vi "Default controls - load control values.vi"(8 "error in (no error)":errorcluster, 11 "path":path) -> (0 "error out":errorcluster, 3 "path to ini":path)   [LabVIEW 2020]
uses:
  Save-Load-Defaults.lvlib/Save-Load-Defaults.lvlib
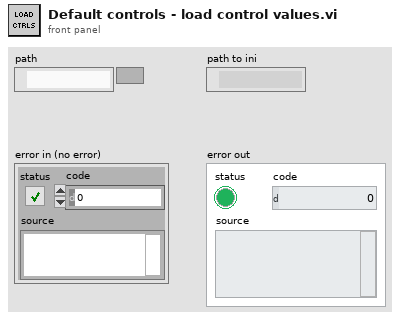
[diagram p1: front panel]
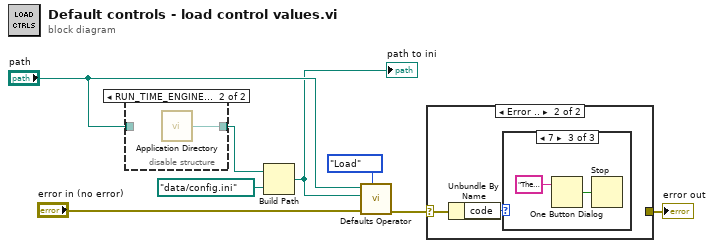
[diagram p0: block diagram]
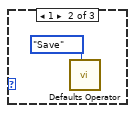
[diagram p4: hidden frame]
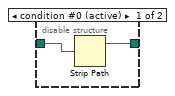
[diagram p5: hidden frame]
diagram:
  n1 = disable-structure shown="RUN_TIME_ENGINE==True" {
    disable-tunnel: "path" -> [w10 _]
    disable-tunnel: [w9 w11] -> w1
    frame condition #0 (active) {
      n2 = Strip Path(path=w10) -> (stripped path=w9:path)  [unwired: 1 out]
    }
    frame condition #1 {
      n3 = call <vilib>:"Application Directory.vi"() -> ("Application Directory"=w11:path)
    }
  }
  n4 = Build Path(base path=w1, name or relative path=path "data/config.ini") -> (appended path=w3:path)
  "path to ini" <- w3
  n5 = call "Defaults Operator.vi"("Operation (Load)"=enum16{"Load", "Save"}."Load", "error in (no error)"="error in (no error)", "INI's path"=w3, "VI's path"="path") -> ("error out"=w7:errorcluster)  [unwired: 5 in, 2 out]
  n6 = case shown="Error .." w7 {
    selector: w7 -> [w12 w14]
    tunnel: [w12 _] -> w8
    frame No Error {
    }
    frame Error {
      n7 = Unbundle By Name(w14) -> ("code"=w13:i32)
      n8 = case shown="7" w13 {
        frame Default {
        }
        frame 1 {
          n9 = call "Defaults Operator.vi"("Operation (Load)"=enum16{"Load", "Save"}."Save") -> ()  [unwired: 8 in, 3 out]
        }
        frame 7 {
          n10 = One Button Dialog(message="The path to INI file or INI format is invalid.\n\nProgram will be quit.\n\n(Error 7)") -> (true=w16:bool)  [unwired: 1 in]
          n11 = Stop(stop? (T)=w16) -> ()
        }
      }
    }
  }
  "error out" <- w8
